vi "ConfigureChannels.vi"(2 "n Channels":i32=8, 3 "input Range (Vpp)":dbl=1.0 format="%.2p", 4 "enable Filter":bool, 5 "ac Coupling":bool) -> (19 "Error Out":errorcluster)   [LabVIEW 2015]
doc: "Configures device parameters for an NI 5170/5171"
uses:
  OscopeAPI/Device Session.lvclass
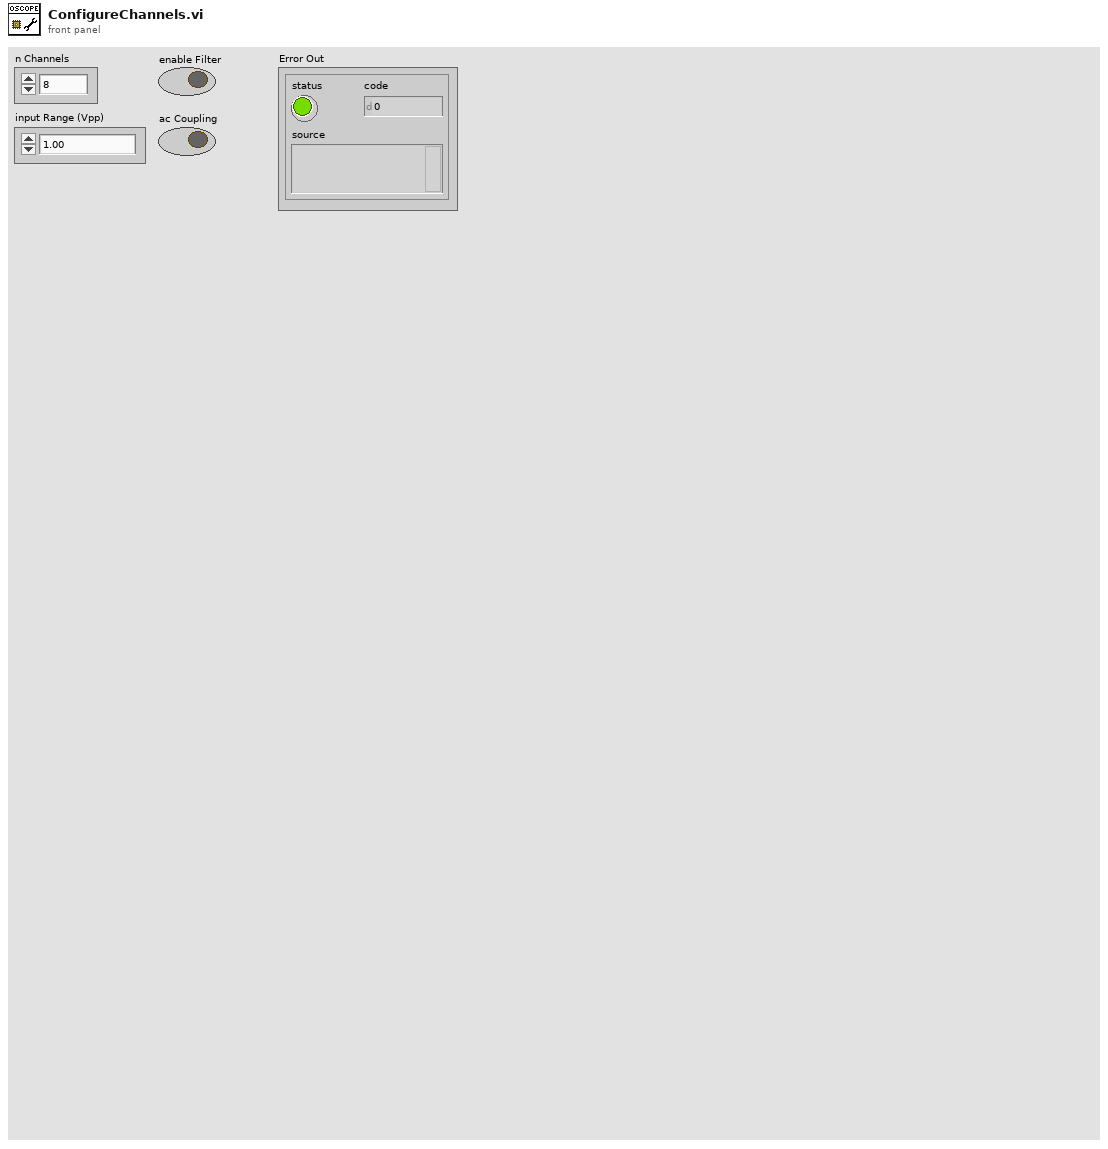
[diagram p1: front panel]
types:
  T1 = enum8{"Default", "Full Bandwidth", "Anti-alias Filter"}
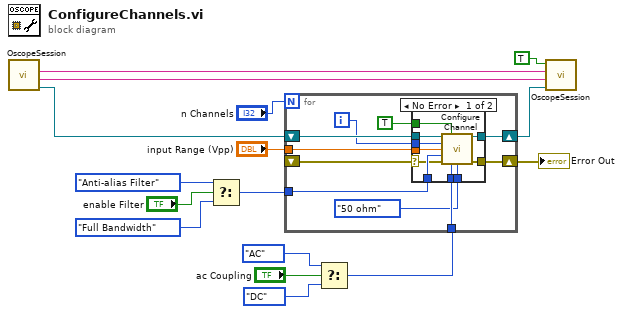
[diagram p0: block diagram]
diagram:
  n1 = call "OscopeSession.vi"() -> ("Session Out"=w1:refnum<class "Device Session.lvclass">, "Bitfile Path Out"=w2:string, "Device Address Out"=w3:string)  [unwired: 9 in]
  n2 = Select(t=T1."Anti-alias Filter" ("Bandwidth"), s="enable Filter", f=T1."Full Bandwidth" ("Bandwidth")) -> (s? t:f=w8:T1)
  n3 = Select(t=enum8{"Default", "DC", "AC"}."AC" ("coupling"), s="ac Coupling", f=enum8{"Default", "DC", "AC"}."DC") -> (s? t:f=w5:enum8{"Default", "DC", "AC"})
  n4 = for {
    N: "n Channels" -> [_]
    shift-right: [w26] -> w15
    shift-left: w1 -> [w24]
    shift-right: [w25] -> w4
    shift-left: _ -> [w17]
    tunnel: "input Range (Vpp)" -> [w22]
    tunnel: w8 -> [w20]
    tunnel: w5 -> [w19]
    i -> [w21]
    n5 = case shown="No Error" w17 {
      selector: w17 -> [w27 w38]
      tunnel: [w36 w37] -> w26
      tunnel: [w35 w38] -> w25
      tunnel: w24 -> [w34 w37]
      tunnel: TRUE ("enable channel") -> [w33 _]
      tunnel: w22 -> [w32 _]
      tunnel: w21 -> [w31 _]
      tunnel: w20 -> [w30 _]
      tunnel: w19 -> [w29 _]
      tunnel: enum8{"Default", "1 mega ohm", "50 ohm"}."50 ohm" ("impedance") -> [w28 _]
      frame No Error {
        n6 = call "Configure Channel.vi"("device session in"=w34, "enable channel (T)"=w33, "channel"=w31, "vertical range (Vpp)"=w32, "bandwidth"=w30, "error in"=w27, "coupling"=w29, "impedance"=w28) -> ("device session out"=w36:refnum<class "Device Session.lvclass">, "error out"=w35:errorcluster)  [unwired: 5 in, 1 out]
      }
      frame Error {
      }
    }
  }
  "Error Out" <- w4
  n7 = call "OscopeSession.vi"("Session In"=w15, "Bitfile Path In"=w2, "Device Address In"=w3, "Write"=TRUE) -> ()  [unwired: 5 in, 3 out]
